vi "Write Section Keys.vi"(6 "Replace? (F)":bool, 7 "Section":string, 8 "error in":errorcluster, 9 "Values":string[](array[string]), 10 "Keys":string[](array[string]), 11 "INI path":path) -> (0 "error out":errorcluster)   [LabVIEW 2017]
uses:
  <vilib>/Utility/config.llb/Write Key (String).vi
  <vilib>/Utility/config.llb/NI_LVConfig.lvlib
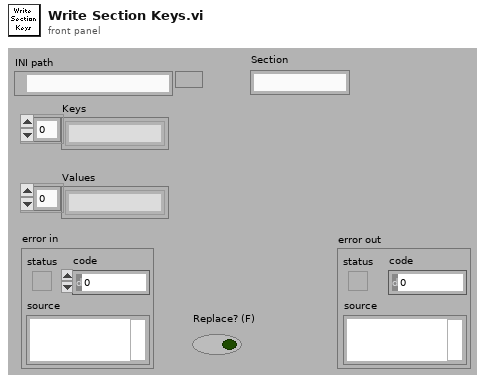
[diagram p1: front panel]
types:
  T1 = typedef "NI_LVConfig.lvlib/Config Data RefNum.ctl" = refnum<k1>
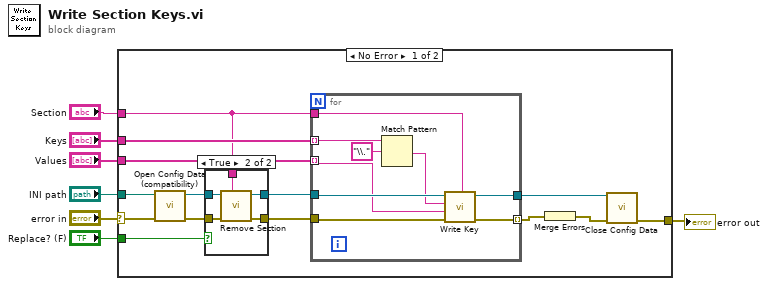
[diagram p0: block diagram]
diagram:
  n1 = case shown="No Error" "error in" {
    selector: "error in" -> [w21 w38]
    tunnel: [w20 w38] -> w6
    tunnel: "INI path" -> [w17 _]
    tunnel: "Section" -> [w9 _]
    tunnel: "Keys" -> [w15 _]
    tunnel: "Values" -> [w14 _]
    tunnel: "Replace? (F)" -> [w8 _]
    frame No Error {
      n2 = call <vilib>:"Open Config Data (compatibility).vi"("error in (no error)"=w21, "configuration file path"=w17) -> ("error out"=w13:errorcluster, "refnum"=w10:T1)  [unwired: 7 in, 1 out]
      n3 = case shown="True" w8 {
        tunnel: w13 -> [w22 w28]
        tunnel: [w22 w27] -> w12
        tunnel: [w23 w26] -> w11
        tunnel: w10 -> [w23 w25]
        tunnel: w9 -> [_ w24]
        frame False {
        }
        frame True {
          n4 = call <vilib>:"Remove Section.vi"("section"=w24, "error in (no error)"=w28, "refnum"=w25) -> ("error out"=w27:errorcluster, "refnum out"=w26:T1)  [unwired: 6 in, 1 out]
        }
      }
      n5 = for {
        tunnel: w12 -> [w37]
        tunnel: [w36] -> w19 mode=indexing
        tunnel: w9 -> [w31]
        tunnel: w11 -> [w35]
        tunnel: [w34] -> w16
        tunnel: w15 -> [w30] mode=indexing
        tunnel: w14 -> [w33] mode=indexing
        n6 = Match Pattern(string=w30, regular expression="\\.") -> (after substring=w29:string)  [unwired: 1 in, 3 out]
        n7 = call-poly <vilib>:"Write Key.vi"("section"=w31, "error in (no error)"=w37, "value"=w33, "key"=w29, "refnum"=w35) -> ("error out"=w36:errorcluster, "refnum out"=w34:T1)  [unwired: 4 in, 1 out]
      }
      n8 = Merge Errors(w19) -> (w18:errorcluster)
      n9 = call <vilib>:"Close Config Data.vi"("error in (no error)"=w18, "refnum"=w16) -> ("error out"=w20:errorcluster)  [unwired: 8 in, 1 out]
    }
    frame Error {
    }
  }
  "error out" <- w6
